vi "PicoScope2000GetValues.vi"(5 "enabled array":i16[](array[numeric]), 7 "Buffer and Transfer Settings":T1 {"Down-Sample Mode" items=["RAW none", "None", "Aggregate", "Decimate", "Average"]; "Down Sample Ratio" step=1; "Samples" format="%_6p"}, 8 "error in (no error)":errorcluster, 10 "Data Pointers In":T2, 11 "handle in":i16) -> (0 "error out":errorcluster, 3 "handle out":i16, 4 "overflow":i16 format="%010b", 6 "noOfSamples":u64)   [LabVIEW 2009]
doc: "Calls ps5000aGetValuesOverlapped"
uses:
  ps2000.dll
  shared/PicoBuffers.ctl
  shared/Buffer and Transfer Settings.ctl
panel:
  out "numSamples":i32
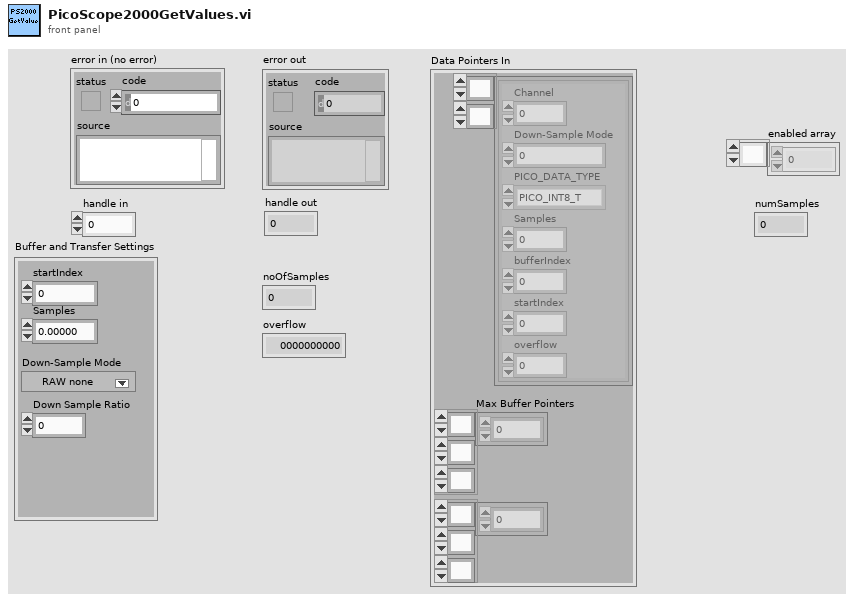
[diagram p1: front panel]
types:
  T1 = typedef "Buffer and Transfer Settings.ctl" = cluster{"startIndex":u64, "Samples":u64, "Down Sample Ratio":u64, "Down-Sample Mode":u32}
  T2 = typedef "PicoBuffers.ctl" = cluster{"Max Buffer Pointers":u64[][][], "Min Buffer Pointers":u64[][][], "StreamingDataInfo":cluster{"Channel":u32, "Down-Sample Mode":u32, "PICO_DATA_TYPE":enum32{"PICO_INT8_T", "PICO_INT16_T", "PICO_INT32_T", "PICO_UINT32_T", "PICO_INT64_T", ""}, "Samples":i32, "bufferIndex":u64, "startIndex":i32, "overflow":i16}[][]}
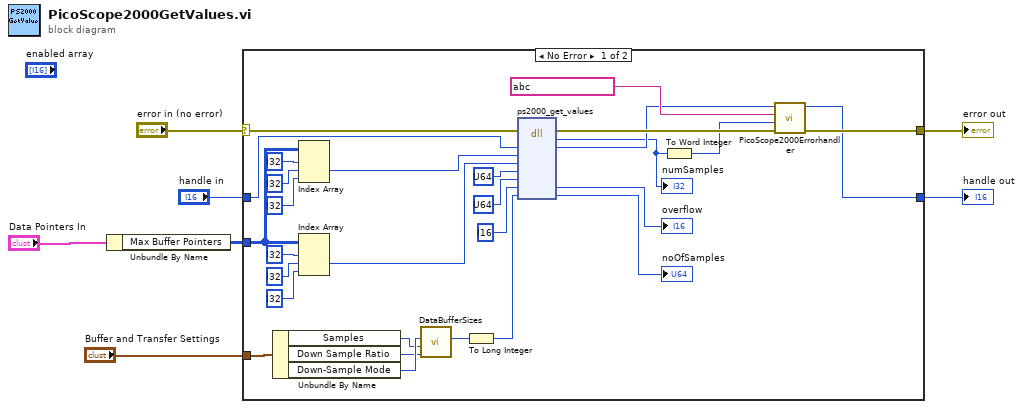
[diagram p0: block diagram]
diagram:
  n1 = Unbundle By Name("Data Pointers In") -> ("Max Buffer Pointers"=w4:u64[][][])
  n2 = case shown="No Error" "error in (no error)" {
    selector: "error in (no error)" -> [w36 w37]
    tunnel: "handle in" -> [w35 w38]
    tunnel: [w10 w38] -> w2
    tunnel: [w14 w37] -> w3
    tunnel: w4 -> [w21 _]
    tunnel: "Buffer and Transfer Settings" -> [w16 _]
    frame #0 {
      n3 = Unbundle By Name(w16) -> ("Samples"=w18:u64, "Down Sample Ratio"=w17:u64, "Down-Sample Mode"=w19:u32)
      n4 = Index Array(array=w21, index (dim 0)=i32 ? ("index (page)"), index (dim 1)=i32 ? ("disabled index (row)"), index (dim 2)=i32 ? ("disabled index (col)")) -> (element=w22:u64)
      n5 = Index Array(array=w21, index (dim 0)=i32 ? ("index (page)"), index (dim 1)=i32 ? ("disabled index (row)"), index (dim 2)=i32 ? ("disabled index (col)")) -> (element=w25:u64)
      n6 = call "DataBufferSizes.vi"("Down Sample Ratio"=w17, "Number of Samples"=w18, "Down-Sample Mode"=w19) -> ("Max Buffer Size"=w15:i32)  [unwired: 7 in, 1 out]
      n7 = To Long Integer(number=w15) -> (32bit integer=w20:i32)
      n8 = dll-call lib="PS2000.dll" fn="ps2000_get_values"(error in=w36, "handle"=w35, "bufferA"=w22, "bufferB"=w25, "bufferC"=u64 ?, "bufferD"=u64 ?, "overflow"=i16 ?, "numValues"=w20) -> (error out=w13:errorcluster, "numSamples"=w8:i32, "handle"=w11:i16, "overflow"=→"overflow":i16, "numValues"=→"noOfSamples":i32)  [unwired: 6 in, 1 out]
      "numSamples" <- w8
      n9 = To Word Integer(number=w8) -> (16bit integer=w9:i16)
      n10 = call "PicoScope2000Errorhandler.vi"("Handle in"=w11, "API function"=string ? ("source"), "Return"=w9, "error in (no error)"=w13) -> ("Handle out"=w10:i16, "error out"=w14:errorcluster)  [unwired: 5 in]
    }
    frame #1 {
    }
  }
  "error out" <- w3
  "handle out" <- w2
